vi "GetDoubleFromDigitalCtrl.vi"(11 "double ref in":refnum<vi>) -> (2 "result":dbl, 3 "double ref out":refnum<vi>)   [LabVIEW 2018, in "Library-Ctrl.lvlib"]
uses:
  Library-Ctrl.lvlib
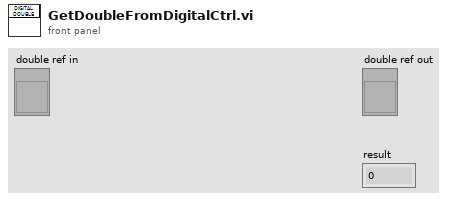
[diagram p1: front panel]
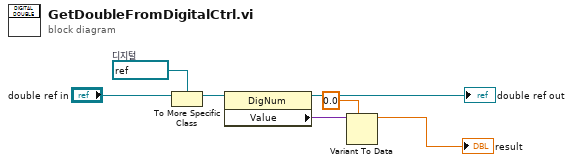
[diagram p0: block diagram]
diagram:
  w6 = refnum<vi> refnum  # 디지털
  n1 = To More Specific Class(target class=w6, reference="double ref in") -> (specific class reference=w5:refnum<vi>)  [unwired: 1 in, 1 out]
  n2 = property class="DigNum"(reference=w5) -> (reference out=→"double ref out":refnum<vi>, "Value"=w4:variant)  [unwired: 1 in, 1 out]
  n3 = Variant To Data(type=0.0, Variant=w4) -> (data=→"result":dbl)  [unwired: 1 in, 1 out]
